vi "DAQNavi Read (Counter 1D Pulse Width NChan 1Samp).vi"(8 "error in (no error)":errorcluster, 11 "task in":i32) -> (0 "error out":errorcluster, 2 "data":cluster{"high period":dbl, "low period":dbl}[](array[cluster]), 3 "task out":i32)   [LabVIEW 2020]
uses:
  DAQNavi_LV.dll
panel:
  in  "timeout":dbl=10.0
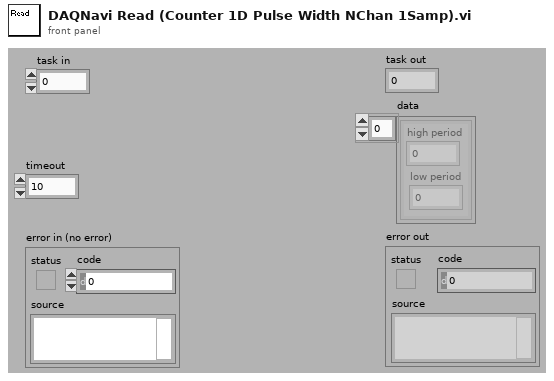
[diagram p1: front panel]
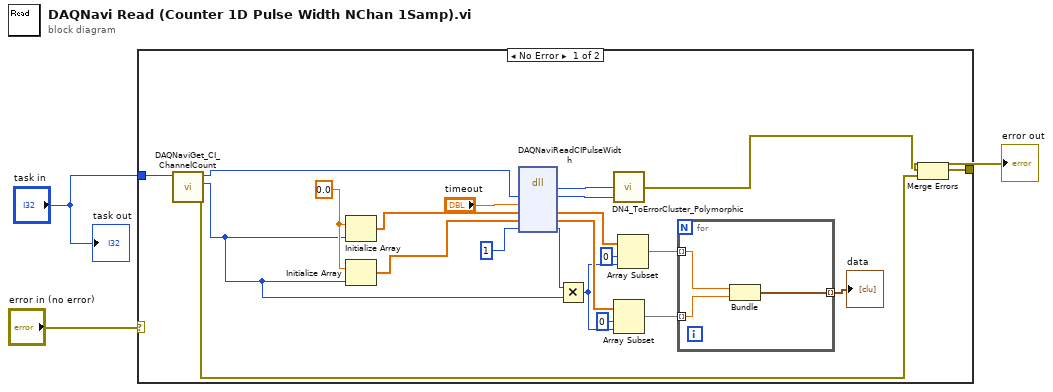
[diagram p0: block diagram]
diagram:
  n1 = case shown="No Error" "error in (no error)" {
    selector: "error in (no error)" -> [_ w29]
    tunnel: "task in" -> [w25 _]
    tunnel: [w6 w29] -> w1
    frame No Error {
      w15 = 0.0 ("element")
      n2 = call "DAQNaviGet_CI_ChannelCount.vi"("task in"=w25) -> ("error out"=w4:errorcluster, "channel count"=w11:i32, "task out"=w16:i32)  [unwired: 1 in, 7 out]
      n3 = Initialize Array(w15, w11) -> (w13:dbl[])
      n4 = Initialize Array(w15, w11) -> (w14:dbl[])
      n5 = dll-call lib="DAQNavi_LV.dll" fn="DAQNaviReadCIPulseWidth"("taskID"=w16, "timeout"="timeout", "hiPeriod"=w13, "loPeriod"=w14, "samples"=u32 1) -> ("return type"=w23:i32, "taskID"=w17:i32, "hiPeriod"=w18:dbl[], "loPeriod"=w20:dbl[], "samples"=w10:u32)  [unwired: 4 in, 2 out]
      n6 = Multiply(x=w10, y=w11) -> (x*y=w12:u32)
      n7 = call "DN4_ToErrorCluster_Polymorphic.vi"("task id"=w17, "error code"=w23) -> ("error out"=w5:errorcluster)  [unwired: 3 out]
      n8 = Array Subset(array=w20, index=0, length=w12) -> (w8:dbl[])
      n9 = Array Subset(array=w18, index=0, length=w12) -> (w9:dbl[])
      n10 = for {
        tunnel: w9 -> [w28] mode=indexing
        tunnel: w8 -> [w27] mode=indexing
        tunnel: [w26] -> w7 mode=indexing
        n11 = Bundle(w28, w27) -> (w26:cluster{dbl, dbl})  [unwired: 1 out]
      }
      "data" <- w7
      n12 = Merge Errors(w5, w4) -> (w6:errorcluster)
    }
    frame Error {
    }
  }
  "error out" <- w1
  "task out" <- "task in"
